vi "Main.vi"() -> ()   [LabVIEW 2015]
doc: "Use this template to build a simple state machine design pattern. Each state executes code and determines which state to transition to."
uses:
  controls/State.ctl
  controls/Data.ctl
panel:
  out "Waveform Chart":dbl[](graph)
  in  "Do Something Else":bool
  in  "Do Smth.":bool caption="Do Something"
  in  "Exit":bool
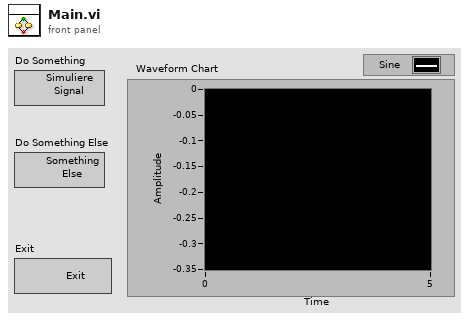
[diagram p1: front panel]
types:
  T1 = typedef "Data.ctl" = cluster{"Boolean":bool, "String":string, "Signal":dbl[]}
  T2 = typedef "State.ctl" = enum16{"Initialize", "Messung simulieren", "Text verknüpfen", "Wait for Event", "User State 2", "Exit"}
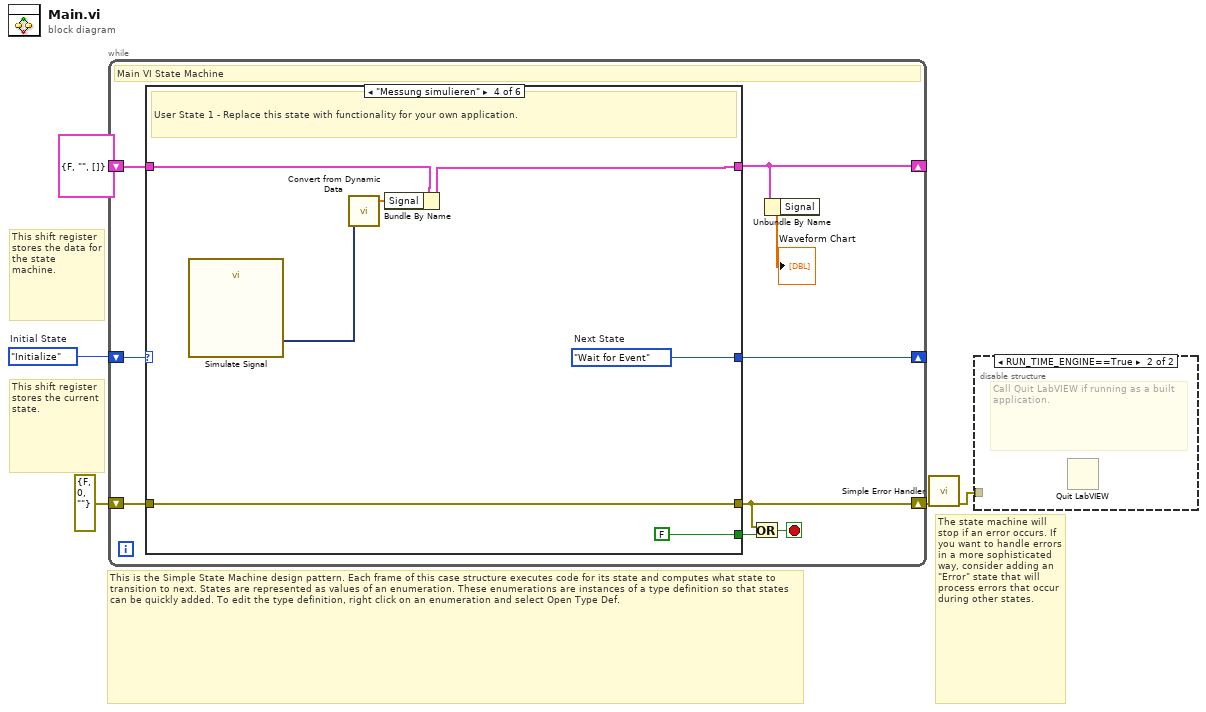
[diagram p0: block diagram]
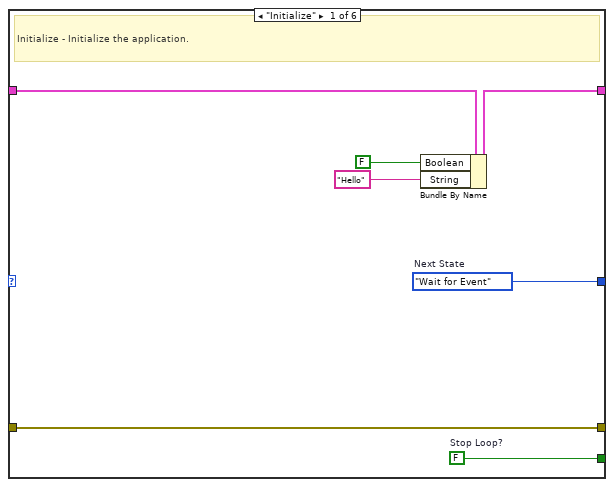
[diagram p3: hidden frame]
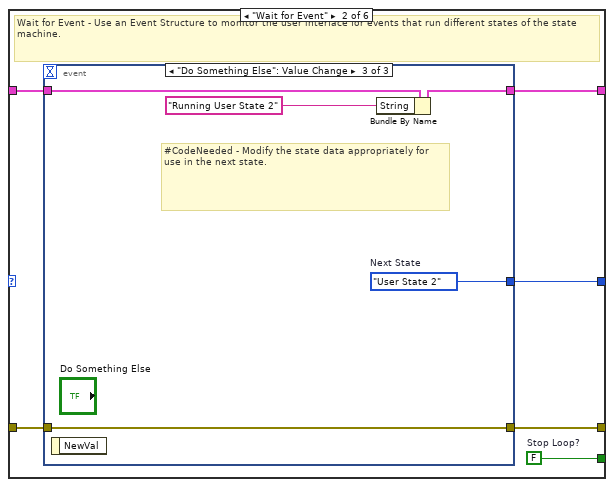
[diagram p4: hidden frame]
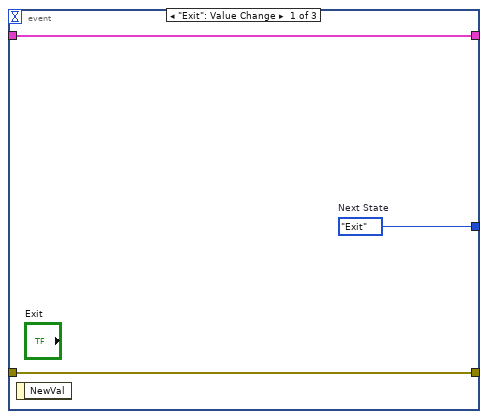
[diagram p5: hidden frame]
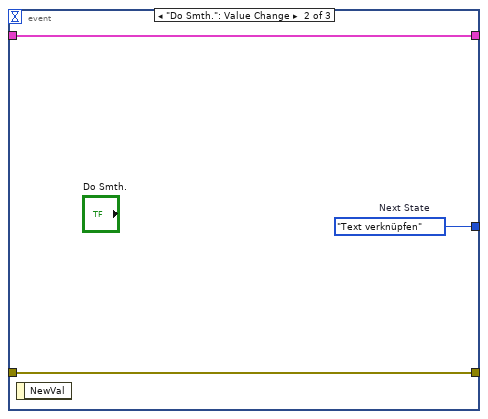
[diagram p6: hidden frame]
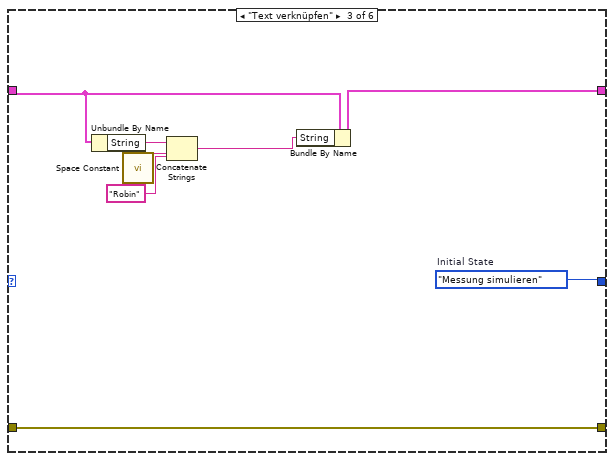
[diagram p7: hidden frame]
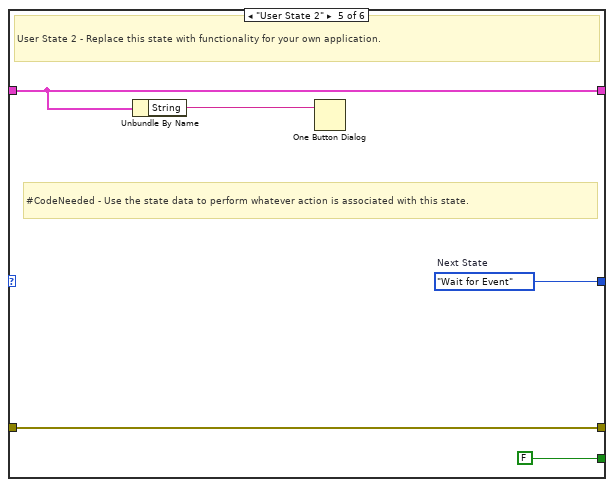
[diagram p8: hidden frame]
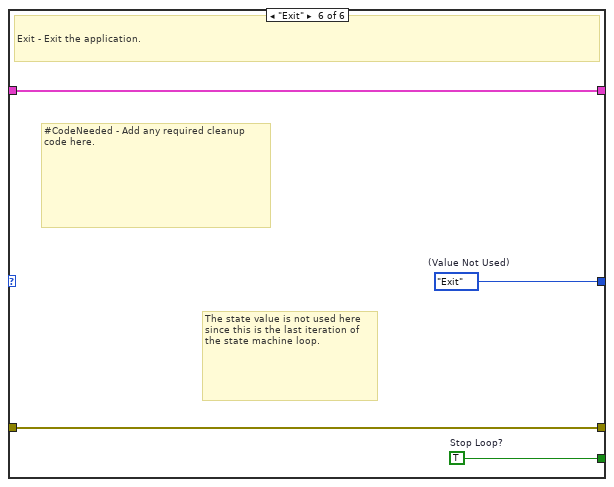
[diagram p9: hidden frame]
diagram:
  w5 = State."Initialize"  # Initial State
  # "The state machine will stop if an error occurs. If you want to handle errors in a more sophisticated way, consider adding an \"Error\" state that will process errors that occur during other states."
  # "This shift register stores the data for the state machine."
  # "This is the Simple State Machine design pattern. Each frame of this case structure executes code for its state and computes what state to transition to next. States are represented as values of an enumeration. These enumerations are instances of a type definition so that states can be quickly added. To edit the type definition, right click on an enumeration and select Open Type Def."
  # "This shift register stores the current state."
  n1 = while {
    shift-right: [w13] -> _
    shift-left: w5 -> [w14]
    shift-right: [w7] -> _
    shift-left: T1 {"Boolean"=FALSE, "String"="", "Signal"=[]} ("Data") -> [w12]
    shift-right: [w8] -> w2
    shift-left: errorcluster {"status"=FALSE, "code"=0, "source"=""} ("error constant") -> [w11]
    stop <- w9 stop-if-true
    # "Main VI State Machine"
    n2 = case shown="\"Messung simulieren\"" w14 {
      tunnel: [w21 w27 w39 w53 w58 w62] -> w13
      tunnel: [w20 w26 _ FALSE ("Stop Loop?") FALSE ("Stop Loop?") w60] -> w10
      tunnel: w12 -> [w19 w25 w42 w50 w56 w61]
      tunnel: [w18 w24 w41 w48 w56 w61] -> w7
      tunnel: w11 -> [w16 w23 w46 w51 w54 w59]
      tunnel: [w16 w22 w46 w51 w54 w59] -> w8
      frame "Initialize" {
        w20 = FALSE  # Stop Loop?
        w21 = State."Wait for Event"  # Next State
        # "Initialize - Initialize the application."
        n3 = Bundle By Name(cluster=w19, "Boolean"=FALSE ("Replace_Me_Boolean"), "String"="Hello") -> (w18:T1)
      }
      frame "Wait for Event" {
        w26 = FALSE  # Stop Loop?
        # "Wait for Event - Use an Event Structure to monitor the user interface for events that run different states of the state machine."
        n4 = event shown="[2] \"Do Something Else\": Value Change" {
          selector: _ -> [_ _ _]
          dyn-events: _ -> [_ _ _]
          timeout: _ -> [_ _ _]
          tunnel: [w30 w33 w38] -> w27
          tunnel: w25 -> [w29 w31 w37]
          tunnel: [w29 w31 w36] -> w24
          tunnel: w23 -> [w28 w32 w34]
          tunnel: [w28 w32 w34] -> w22
          event "Exit": Value Change {
            w30 = State."Exit"  # Next State
            n5 = event-data() -> ()  [unwired: 1 in, 1 out]
          }
          event "Do Smth.": Value Change {
            w33 = State."Text verknüpfen"  # Next State
            n6 = event-data() -> ()  [unwired: 1 in, 1 out]
          }
          event "Do Something Else": Value Change {
            w38 = State."User State 2"  # Next State
            # "#CodeNeeded - Modify the state data appropriately for use in the next state."
            n7 = event-data() -> ()  [unwired: 1 in, 1 out]
            n8 = Bundle By Name(cluster=w37, "String"="Running User State 2" ("Running User State 2")) -> (w36:T1)
          }
        }
      }
      frame "Text verknüpfen" {
        w39 = State."Messung simulieren"  # Initial State
        n9 = Unbundle By Name(w42) -> ("String"=w45:string)
        n10 = call <vilib>:"Space Constant.vi"() -> ("String"=w43:string)
        n11 = Concatenate Strings(w45, w43, "Robin" ("string")) -> (w40:string)
        n12 = Bundle By Name(cluster=w42, "String"=w40) -> (w41:T1)
      }
      frame "Messung simulieren" {
        w53 = State."Wait for Event"  # Next State
        # "User State 1 - Replace this state with functionality for your own application."
        n13 = call "Simulate Signal"() -> ("Sine"=w47:dynamicdata)  [unwired: 14 in, 1 out]
        n14 = call "Convert from Dynamic Data"("Dynamic Data Type"=w47) -> ("Array"=w49:dbl[])  [unwired: 3 in]
        n15 = Bundle By Name(cluster=w50, "Signal"=w49) -> (w48:T1)
      }
      frame "User State 2" {
        w58 = State."Wait for Event"  # Next State
        # "#CodeNeeded - Use the state data to perform whatever action is associated with this state."
        # "User State 2 - Replace this state with functionality for your own application."
        n16 = Unbundle By Name(w56) -> ("String"=w55:string)
        n17 = One Button Dialog(message=w55) -> ()  [unwired: 1 in, 1 out]
      }
      frame "Exit" {
        w60 = TRUE  # Stop Loop?
        w62 = State."Exit"  # (Value Not Used)
        # "#CodeNeeded - Add any required cleanup code here."
        # "The state value is not used here since this is the last iteration of the state machine loop."
        # "Exit - Exit the application."
      }
    }
    n18 = Or(x=w8, y=w10) -> (x .or. y?=w9:bool)
    n19 = Unbundle By Name(w7) -> ("Signal"=→"Waveform Chart":dbl[])
  }
  n20 = call <vilib>:"Simple Error Handler.vi"("error in (no error)"=w2) -> ("error out"=w1:errorcluster)  [unwired: 4 in, 4 out]
  n21 = disable-structure shown="RUN_TIME_ENGINE==True" {
    disable-tunnel: w1 -> [_ _]
    frame condition #0 (active) {
    }
    frame condition #1 {
      # "Call Quit LabVIEW if running as a built application."
      n22 = Quit LabVIEW() -> ()  [unwired: 1 in]
    }
  }
